vi "SerialTest.vi"() -> ()   [LabVIEW 2009, in "Test.lvlib"]
uses:
  Test.lvlib
  Serial.lvlib
panel:
  out "is Timeout":bool
  out "is Corrupted":bool
  out "data out":u8[](array[numeric])
  out "Message ID Out":u32 format="%x"
  in  "data":u8[](array[numeric])
  in  "messageID":u32 format="%.0x"
  out "error out":errorcluster
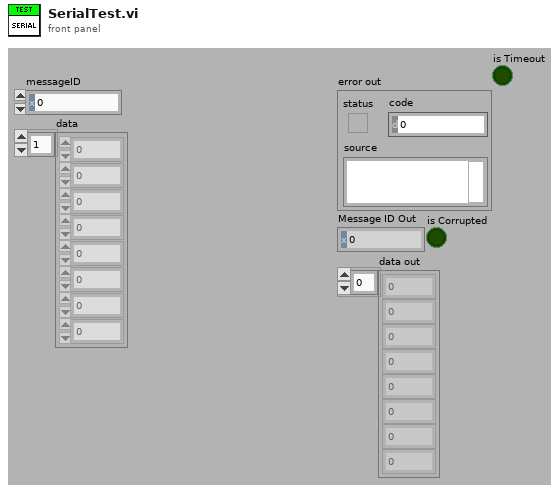
[diagram p1: front panel]
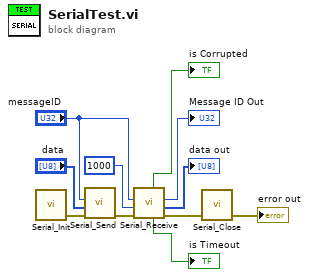
[diagram p0: block diagram]
diagram:
  n1 = call "Serial_Init.vi"() -> ("error out"=w11:errorcluster)  [unwired: 4 in, 1 out]
  n2 = call "Serial_Send.vi"("error in"=w11, "data"="data", "messageID"="messageID") -> ("error out"=w9:errorcluster)  [unwired: 7 in, 1 out]
  n3 = call "Serial_Receive.vi"("error in (no error)"=w9, "timeoutMs"=u32 1000, "Message ID"="messageID") -> ("error out"=w8:errorcluster, "data"=→"data out":u8[], "Message ID Out"=→"Message ID Out":u32, "is Timeout"=→"is Timeout":bool, "is Corrupted"=→"is Corrupted":bool)  [unwired: 3 in, 1 out]
  n4 = call "Serial_Close.vi"("error in (no error)"=w8) -> ("error out"=→"error out":errorcluster)  [unwired: 4 in]
